vi "json Insert U32 - string path.vi"(8 "error in (no error)":errorcluster, 9 "anything":u32, 10 "path":string, 11 "JSON Document in":refnum<class "JSON Document.lvclass">) -> (0 "error out":errorcluster, 1 "replaced?":bool, 3 "JSON Document out":refnum<class "JSON Document.lvclass">)   [LabVIEW 2015, in "JSON Document.lvclass"]
uses:
  JSON Document.lvclass
  JSON Document.lvclass/JSON Document.ctl
  rapidjson wrapper/rapidjson wrapper.lvlib
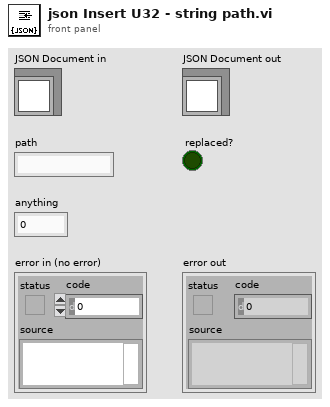
[diagram p1: front panel]
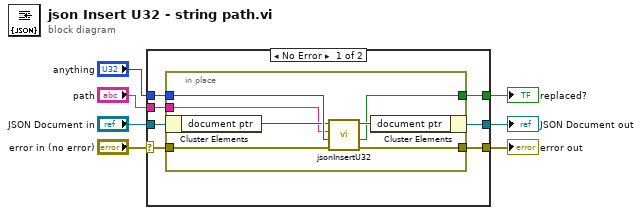
[diagram p0: block diagram]
diagram:
  n1 = case shown="No Error" "error in (no error)" {
    selector: "error in (no error)" -> [w10 w23]
    tunnel: [w11 w23] -> w6
    tunnel: [w13 w22] -> w4
    tunnel: "JSON Document in" -> [w14 w22]
    tunnel: "anything" -> [w9 _]
    tunnel: "path" -> [w12 _]
    tunnel: [w8 _] -> w1
    frame No Error {
      n2 = in-place {
        in-place-border: w12 -> [w16]
        in-place-border: w10 -> [w20]
        in-place-border: [w19] -> w11
        in-place-border: w9 -> [w18]
        in-place-border: [w15] -> w8
        n3 = in-place-cluster #1(w14) -> ("document ptr"=w17:i64)
        n4 = call "jsonInsertU32.vi"("error in (no error)"=w20, "value"=w18, "path"=w16, "d in"=w17) -> ("error out"=w19:errorcluster, "replaced?"=w15:bool, "d out"=w21:i64)  [unwired: 5 in]
        n5 = in-place-cluster #1("document ptr"=w21) -> (w13:refnum<class "JSON Document.lvclass">)
      }
    }
    frame Error {
    }
  }
  "error out" <- w6
  "JSON Document out" <- w4
  "replaced?" <- w1
